vi "AcquirerWithAI.vi"(0 "waveform data":T3, 11 "command stream":T4) -> (1 "status stream":T5, 2 "wfm data lossy stream":T6, 3 "done":bool=TRUE, 4 "start/stop":T1, 5 "wfm data stream":T3, 6 "settings":T2, 7 "file path tag":T7, 8 "exit":T1)   [LabVIEW 2019]
uses:
  <extravilib>/ChannelInstances/Tag-path/))Channel.ctl
  <extravilib>/ChannelInstances/Stream-a[.](wfm(dbl))/)Channel.ctl
  <extravilib>/ChannelInstances/Lossy Stream-a[.](wfm(dbl))/)Channel.ctl
  <extravilib>/ChannelInstances/Stream-str/)Channel.ctl
  <resource>/Channels/Messenger/))Channel.ctl
  <vilib>/ChannelSupport/Channel Message/Channel Message.lvclass
  <extravilib>/ChannelInstances/Tag-t'Measure and Log Settings.ctl'/))Channel.ctl
  subVIs/Measure and Log Settings.ctl
  subVIs/Simulated Signal Type.ctl
  <extravilib>/ChannelInstances/Tag-bool/))Channel.ctl
  messages/MeasureAndLogMessage.lvclass/MeasureAndLogMessage.ctl
  <resource>/Channels/Messenger/Read With Abort.vi
  <vilib>/ChannelSupport/Channel Message/Read ID.vi
  <extravilib>/ChannelInstances/Stream-a[.](wfm(dbl))/Read With Abort.vi
  <extravilib>/ChannelInstances/Stream-a[.](wfm(dbl))/Endpoint.vi
  <extravilib>/ChannelInstances/Stream-a[.](wfm(dbl))/EndpointRead.vi
  <extravilib>/ChannelInstances/Lossy Stream-a[.](wfm(dbl))/Endpoint.vi
  <extravilib>/ChannelInstances/Stream-str/Endpoint.vi
  <resource>/Channels/Messenger/Endpoint.vi
  <extravilib>/ChannelInstances/Tag-t'Measure and Log Settings.ctl'/Endpoint.vi
  <extravilib>/ChannelInstances/Tag-path/Endpoint.vi
  <extravilib>/ChannelInstances/Tag-bool/Endpoint.vi
  <extravilib>/ChannelInstances/Stream-a[.](wfm(dbl))/)Channel.vi
  <resource>/ChannelSupport/_ChannelSupport/WaitIfNeeded.vi
  <extravilib>/ChannelInstances/Lossy Stream-a[.](wfm(dbl))/)Channel.vi
  <extravilib>/ChannelInstances/Stream-str/)Channel.vi
  messages/MeasureAndLogMessage.lvclass
  <resource>/Channels/Messenger/Messenger.lvlib
  <extravilib>/ChannelInstances/Stream-a[.](wfm(dbl)).lvlib
  <extravilib>/ChannelInstances/Tag-path.lvlib
  <extravilib>/ChannelInstances/Tag-t'Measure and Log Settings.ctl'.lvlib
  <extravilib>/ChannelInstances/Tag-bool.lvlib
  <extravilib>/ChannelInstances/Stream-str.lvlib
  <extravilib>/ChannelInstances/Lossy Stream-a[.](wfm(dbl)).lvlib
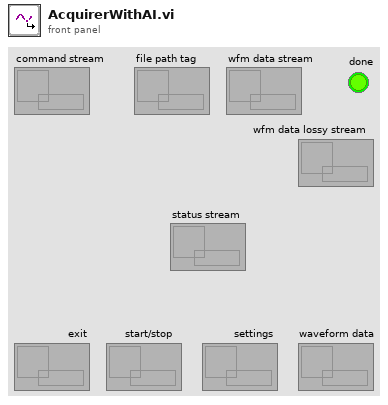
[diagram p1: front panel]
types:
  T1 = typedef "Tag-bool.lvlib/))Channel.ctl" = refnum<queue>
  T2 = typedef "Tag-t'Measure and Log Settings.ctl'.lvlib/))Channel.ctl" = refnum<queue>
  T3 = typedef "Stream-a[.](wfm(dbl)).lvlib/)Channel.ctl" = refnum<queue>
  T4 = typedef "Messenger.lvlib/))Channel.ctl" = refnum<queue>
  T5 = typedef "Stream-str.lvlib/)Channel.ctl" = refnum<queue>
  T6 = typedef "Lossy Stream-a[.](wfm(dbl)).lvlib/)Channel.ctl" = refnum<queue>
  T7 = typedef "Tag-path.lvlib/))Channel.ctl" = refnum<queue>
  T8 = typedef "Measure and Log Settings.ctl" = cluster{"sample rate":dbl, "input range":dbl, "logfile path":path, "Simulated Signal":cluster{"signal type":T9, "frequency":dbl, "amplitude":dbl}}
  T9 = typedef "Simulated Signal Type.ctl" = enum16{"Sine Wave", "Square Wave with Noise"}
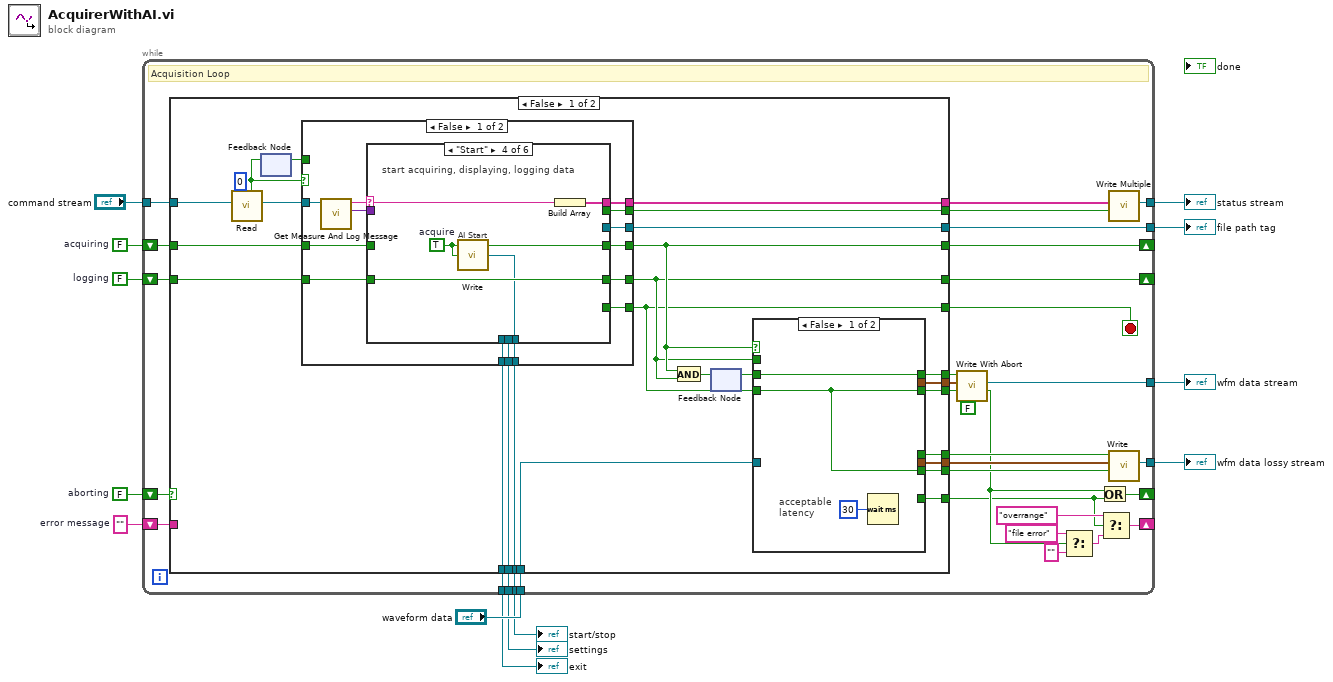
[diagram p0: block diagram]
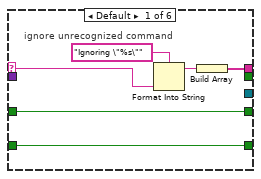
[diagram p2: hidden frame]
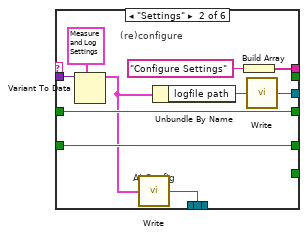
[diagram p3: hidden frame]
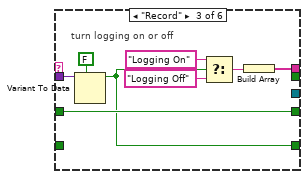
[diagram p4: hidden frame]
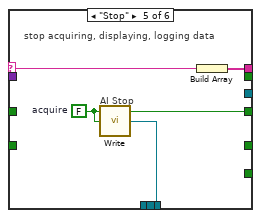
[diagram p5: hidden frame]
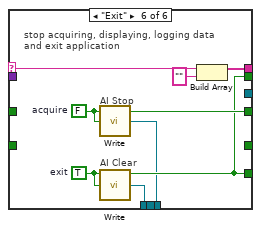
[diagram p6: hidden frame]
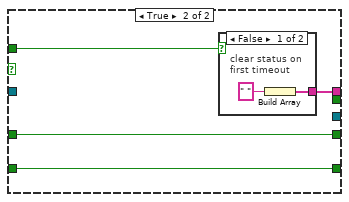
[diagram p7: hidden frame]
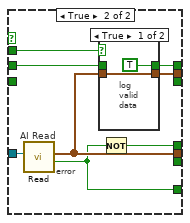
[diagram p9: hidden frame]
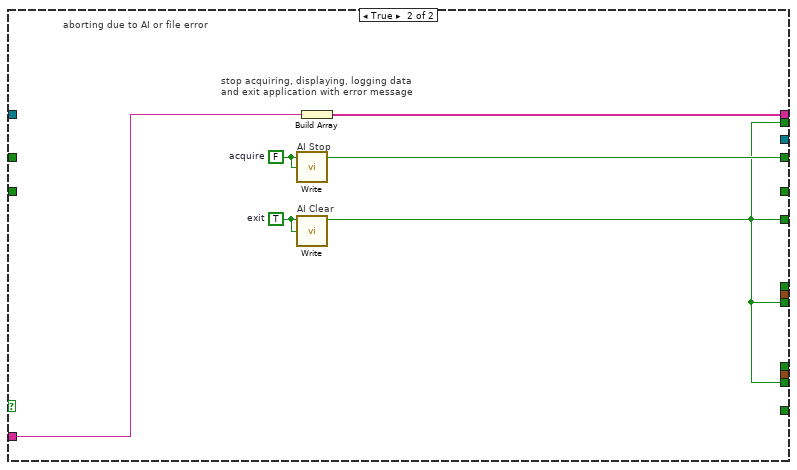
[diagram p11: hidden frame]
diagram:
  w9 = ""  # error message
  w8 = FALSE  # aborting
  w7 = FALSE  # logging
  w6 = FALSE  # acquiring
  n1 = while {
    tunnel: "command stream" -> [w45]
    tunnel: [w37] -> w10
    tunnel: [w34] -> w11
    tunnel: [w30] -> w12
    shift-right: [w42] -> _
    shift-left: w6 -> [w43]
    shift-right: [w41] -> _
    shift-left: w7 -> [w46]
    tunnel: [w44] -> w13
    shift-right: [w29] -> _
    shift-left: w8 -> [w40]
    shift-right: [w20] -> _
    shift-left: w9 -> [w39]
    tunnel: [w17] -> w2
    tunnel: [w16] -> w3
    tunnel: [w15] -> w1
    tunnel: "waveform data" -> [w14]
    stop <- w38 stop-if-true
    # "Acquisition Loop"
    n2 = case shown="False" w40 {
      tunnel: w46 -> [w72 _]
      tunnel: w45 -> [w71 _]
      tunnel: [w66 _] -> w44
      tunnel: w43 -> [w65 _]
      tunnel: [w64 w150] -> w42
      tunnel: [w63 _] -> w41
      tunnel: [w60 w147] -> w38
      tunnel: w39 -> [_ w149]
      tunnel: [w58 w147] -> w36
      tunnel: [w59 w148] -> w35
      tunnel: [w56 w147] -> w33
      tunnel: [w57 _] -> w32
      tunnel: [w55 _] -> w31
      tunnel: [w54 _] -> w21
      tunnel: [w53 _] -> w28
      tunnel: [w52 w147] -> w27
      tunnel: [w51 _] -> w26
      tunnel: [w50 _] -> w17
      tunnel: [w49 _] -> w16
      tunnel: [w48 _] -> w15
      tunnel: w14 -> [w47 _]
      frame False {
        n3 = call <extravilib>:"Read.vi"("timeout in ms (-1)"=0, "channel"=w71) -> ("element"=w70:refnum<class "Channel Message.lvclass">, "timed out?"=w68:bool)  [unwired: 7 in, 1 out]
        n4 = feedback #1() -> (w67:bool)  [unwired: 1 in]
        n5 = feedback-in #1(w68) -> ()
        n6 = case shown="False" w68 {
          tunnel: w70 -> [w86 _]
          tunnel: [w83 _] -> w60
          tunnel: [w82 w130] -> w64
          tunnel: w65 -> [w81 w130]
          tunnel: [w80 w129] -> w63
          tunnel: w72 -> [w79 w129]
          tunnel: w67 -> [_ w128]
          tunnel: [w78 _] -> w66
          tunnel: [w77 w127] -> w59
          tunnel: [w76 _] -> w58
          tunnel: [w75 _] -> w50
          tunnel: [w74 _] -> w49
          tunnel: [w73 _] -> w48
          frame False {
            n7 = call "Get Measure And Log Message.vi"("MyMessage"=w86) -> ("args"=w84:variant, "command"=w85:string)  [unwired: 7 in, 2 out]
            n8 = case shown="\"Start\"" w85 {
              selector: w85 -> [w92 _ _ w113 w118 w126]
              tunnel: w84 -> [_ w100 w109 _ _ _]
              tunnel: [_ _ _ _ _ w122] -> w83
              tunnel: [w90 w102 w110 w115 w119 w124] -> w82
              tunnel: w81 -> [w90 w102 w110 _ _ _]
              tunnel: [w89 w101 w105 w114 _ _] -> w80
              tunnel: w79 -> [w89 w101 _ w114 _ _]
              tunnel: [_ w97 _ _ _ _] -> w78
              tunnel: [w87 w94 w103 w112 w117 w123] -> w77
              tunnel: [_ _ _ _ _ w122] -> w76
              tunnel: [_ _ _ w111 w116 w121] -> w75
              tunnel: [_ _ _ _ _ w120] -> w74
              tunnel: [_ w93 _ _ _ _] -> w73
              frame Default {
                # "ignore unrecognized command"
                n9 = Format Into String(format string="Ignoring \"%s\"", w92) -> (resulting string=w88:string)  [unwired: 2 in, 1 out]
                n10 = Build Array(w88) -> (w87:string[])
              }
              frame "Settings" {
                # "AI Config"
                # "(re)configure"
                n11 = Variant To Data(type=T8 {"sample rate"=100.0, "input range"=10.0, "logfile path"=path "/Volumes/Bohr/Users/jeffk/Documents/LabVIEW Data/Logged Data.tdms", "Simulated Signal"={"signal type"=enum."Sine Wave", "frequency"=1000.0, "amplitude"=5.0}} ("settings out"), Variant=w100) -> (data=w99:T8)  [unwired: 1 in, 1 out]
                n12 = call <extravilib>:"Write.vi"("element"=w99) -> ("channel"=w93:T2)  [unwired: 1 out]
                n13 = Unbundle By Name(w99) -> ("logfile path"=w98:path)
                n14 = Build Array("Configure Settings" ("element")) -> (w94:string[])
                n15 = call <extravilib>:"Write.vi"("element"=w98) -> ("channel"=w97:T7)  [unwired: 1 out]
              }
              frame "Record" {
                # "turn logging on or off"
                n16 = Variant To Data(type=FALSE, Variant=w109) -> (data=w105:bool)  [unwired: 1 in, 1 out]
                n17 = Select(t="Logging On", s=w105, f="Logging Off") -> (s? t:f=w104:string)
                n18 = Build Array(w104) -> (w103:string[])
              }
              frame "Start" {
                w115 = TRUE  # acquire
                # "AI Start"
                # "start acquiring, displaying, logging data"
                n19 = call <extravilib>:"Write.vi"("element"=w115) -> ("channel"=w111:T1)  [unwired: 1 out]
                n20 = Build Array(w113) -> (w112:string[])
              }
              frame "Stop" {
                w119 = FALSE  # acquire
                # "AI Stop"
                # "stop acquiring, displaying, logging data"
                n21 = call <extravilib>:"Write.vi"("element"=w119) -> ("channel"=w116:T1)  [unwired: 1 out]
                n22 = Build Array(w118) -> (w117:string[])
              }
              frame "Exit" {
                w124 = FALSE  # acquire
                w122 = TRUE  # exit
                # "AI Clear"
                # "AI Stop"
                # "stop acquiring, displaying, logging data\nand exit application"
                n23 = call <extravilib>:"Write.vi"("element"=w124) -> ("channel"=w121:T1)  [unwired: 1 out]
                n24 = call <extravilib>:"Write.vi"("element"=w122) -> ("channel"=w120:T1)  [unwired: 1 out]
                n25 = Build Array(w126, "" ("element")) -> (w123:string[])
              }
            }
          }
          frame True {
            n26 = case shown="False" w128 {
              tunnel: [w131 _] -> w127
              frame False {
                # "clear status on\nfirst timeout"
                n27 = Build Array(" " ("string")) -> (w131:string[])
              }
              frame True {
              }
            }
          }
        }
        n28 = And(x=w64, y=w63) -> (x .and. y?=w62:bool)
        n29 = feedback #2() -> (w61:bool)  [unwired: 1 in]
        n30 = feedback-in #2(w62) -> ()
        n31 = case shown="False" w64 {
          tunnel: w63 -> [_ w143]
          tunnel: w61 -> [w135 w142]
          tunnel: w60 -> [w134 _]
          tunnel: [_ w140] -> w57
          tunnel: [w134 _] -> w56
          tunnel: [_ w141] -> w55
          tunnel: [_ w137] -> w54
          tunnel: [w135 w138] -> w53
          tunnel: [w134 _] -> w52
          tunnel: [_ w139] -> w51
          tunnel: w47 -> [_ w136]
          frame False {
            # "acceptable\nlatency"
            n32 = Wait (ms)(milliseconds to wait=u32 30) -> ()  [unwired: 1 out]
          }
          frame True {
            # "error"
            # "AI Read"
            n33 = call <extravilib>:"Read.vi"("channel"=w136) -> ("last element?"=w137:bool, "element"=w141:waveform(dbl)[])  [unwired: 6 in, 3 out]
            n34 = case shown="True" w143 {
              tunnel: w141 -> [w145 _]
              tunnel: w142 -> [_ w146]
              tunnel: [w145 _] -> w139
              tunnel: [TRUE w146] -> w138
              frame True {
                # "log \nvalid\ndata"
              }
              frame False {
              }
            }
            n35 = Not(x=w137) -> (.not. x?=w140:bool)
          }
        }
      }
      frame True {
        w150 = FALSE  # acquire
        w147 = TRUE  # exit
        # "aborting due to AI or file error"
        # "AI Clear"
        # "AI Stop"
        # "stop acquiring, displaying, logging data\nand exit application with error message"
        n36 = call <extravilib>:"Write.vi"("element"=w150) -> ()  [unwired: 2 out]
        n37 = call <extravilib>:"Write.vi"("element"=w147) -> ()  [unwired: 2 out]
        n38 = Build Array(w149) -> (w148:string[])
      }
    }
    n39 = call <extravilib>:"Write With Abort.vi"("abort"=FALSE, "last element? (F)"=w27, "element"=w26, "element valid? (T)"=w28) -> ("aborted?"=w24:bool, "channel"=w30:T3)  [unwired: 4 in, 2 out]
    n40 = Select(t="file error", s=w24, f="") -> (s? t:f=w19:string)
    n41 = Or(x=w24, y=w21) -> (x .or. y?=w29:bool)
    n42 = Select(t="overrange", s=w21, f=w19) -> (s? t:f=w20:string)
    n43 = call <extravilib>:"Write Multiple.vi"("last element? (F)"=w36, "elements"=w35) -> ("channel"=w37:T5)  [unwired: 6 in, 3 out]
    n44 = call <extravilib>:"Write.vi"("last element? (F)"=w33, "element"=w31, "element valid? (T)"=w32) -> ("channel"=w34:T6)  [unwired: 6 in, 2 out]
  }
  "file path tag" <- w13
  "wfm data stream" <- w12
  "wfm data lossy stream" <- w11
  "status stream" <- w10
  "start/stop" <- w2
  "exit" <- w3
  "settings" <- w1
